vi "GDSLvClass_FlattenClass.vi"(0 "Class Refnum In":refnum<vi>, 3 "FlattenClass(T=>Flat,F=>Not Flat)":bool, 5 "error in (no error)":errorcluster) -> (14 "Class Refnum Out":refnum<vi>, 19 "error out":errorcluster)   [LabVIEW 2020]
panel:
  out "FoldersToActOn(Empty=>AllFolders) 2":string[](array[string])
  in  "FoldersToActOn(Empty=>AllFolders)":string[](array[string])
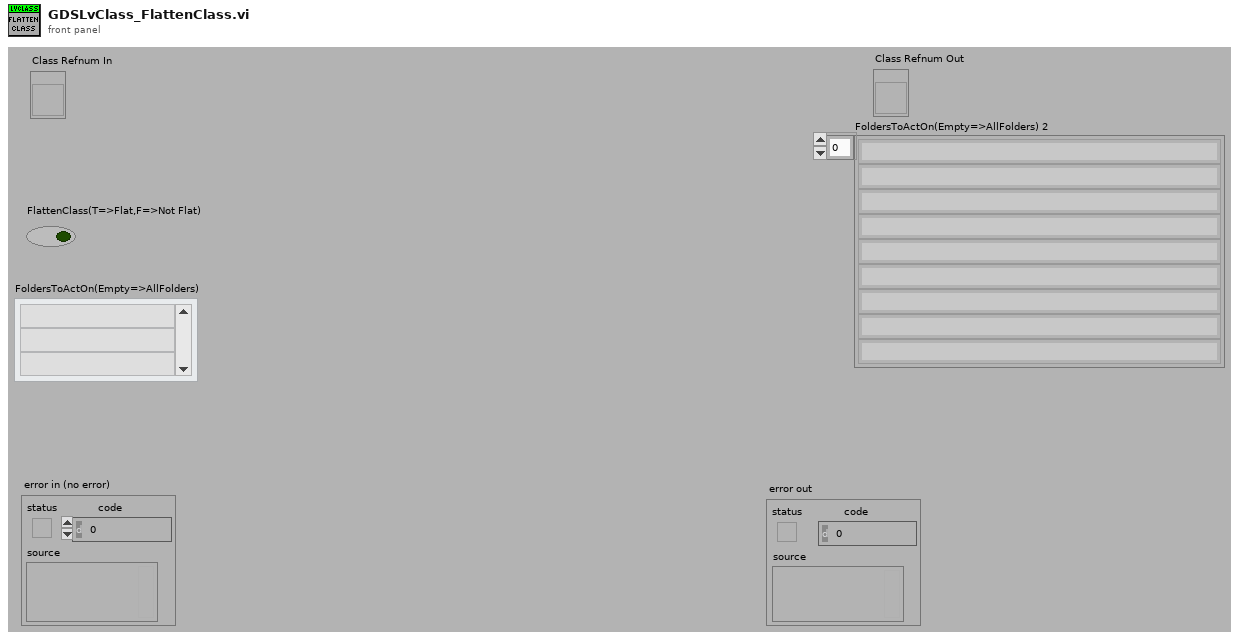
[diagram p1: front panel]
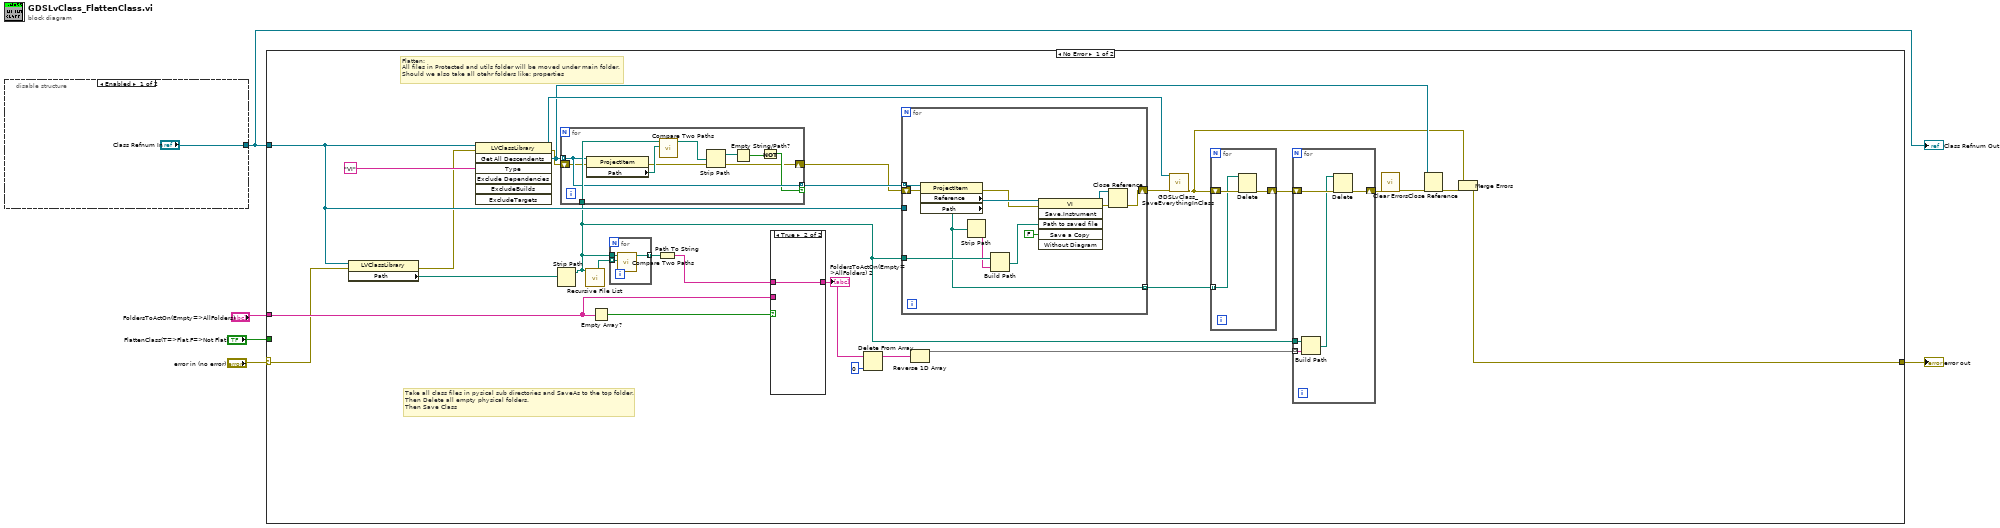
[diagram p0: block diagram]
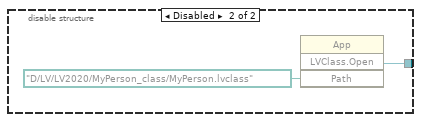
[diagram p2: hidden frame]
diagram:
  n1 = disable-structure shown="Enabled" {
    disable-tunnel: ["Class Refnum In" w8] -> w3
    frame Enabled {
    }
    frame Disabled {
      n2 = invoke class="App" method="LVClass.Open"("Path"=path "D:/LV/LV2020/MyPerson_class/MyPerson.lvclass") -> ("LVClass.Open"=w8:refnum<vi>)  [unwired: 3 in, 3 out]
    }
  }
  "Class Refnum Out" <- w3
  n3 = case shown="No Error" "error in (no error)" {
    selector: "error in (no error)" -> [w25 w71]
    tunnel: [w9 w71] -> w4
    tunnel: w3 -> [w28 _]
    tunnel: "FlattenClass(T=>Flat,F=>Not Flat)" -> [_ _]
    tunnel: "FoldersToActOn(Empty=>AllFolders)" -> [w33 _]
    frame No Error {
      # "Take all class files in pysical sub directories and SaveAs to the top folder.\nThen Delete all empty physical folders.\nThen Save Class"
      # "Flatten:\nAll files in Protected and utils folder will be moved under main folder.\nShould we also take all otehr folders like: properties"
      n4 = property class="LVClassLibrary"(reference=w28, error in=w25) -> (error out=w24:errorcluster, "Path"=w35:path)  [unwired: 1 out]
      n5 = invoke class="LVClassLibrary" method="Get All Descendents"(reference=w28, error in=w24, "Type"="VI") -> (reference out=w22:refnum<vi>, error out=w26:errorcluster, "All Descendents"=w12:refnum<vi>[])  [unwired: 4 in, 4 out]
      n6 = Strip Path(path=w35) -> (stripped path=w16:path)  [unwired: 1 out]
      n7 = for {
        tunnel: w12 -> [w60] mode=indexing
        tunnel: w16 -> [w65]
        tunnel: [w60] -> w29 mode=indexing if=w59
        shift-right: [w58] -> w27
        shift-left: w26 -> [w57]
        n8 = property class="ProjectItem"(reference=w60, error in=w57) -> (error out=w58:errorcluster, "Path"=w64:path)  [unwired: 1 out]
        n9 = call <vilib>:"Compare Two Paths.vi"("Path 2"=w64, "Path 1"=w65) -> ("Relative Path from 1 to 2"=w63:path)  [unwired: 6 in, 3 out]
        n10 = Strip Path(path=w63) -> (stripped path=w62:path)  [unwired: 1 out]
        n11 = Empty String/Path?(string/path=w62) -> (empty?=w61:bool)
        n12 = Not(x=w61) -> (.not. x?=w59:bool)
      }
      n13 = call <vilib>:"Recursive File List.vi"("Folder Path"=w16) -> ("All Folders"=w30:path[])  [unwired: 6 in, 4 out]
      n14 = Empty Array?(array=w33) -> (empty?=w34:bool)
      n15 = for {
        tunnel: w16 -> [w68]
        tunnel: w30 -> [w67] mode=indexing
        tunnel: [w66] -> w32 mode=indexing
        n16 = call <vilib>:"Compare Two Paths.vi"("Path 2"=w67, "Path 1"=w68) -> ("Relative Path from 1 to 2"=w66:path)  [unwired: 6 in, 3 out]
      }
      n17 = Path To String(path=w32) -> (string=w31:string[])
      n18 = case shown="True" w34 {
        tunnel: w31 -> [_ w70]
        tunnel: [w69 w70] -> w20
        tunnel: w33 -> [w69 _]
        frame False {
        }
        frame True {
        }
      }
      "FoldersToActOn(Empty=>AllFolders) 2" <- w20
      n19 = Delete From Array(array=w20, index=0) -> (array with subset deleted=w17:string[])  [unwired: 1 in, 1 out]
      n20 = for {
        tunnel: w29 -> [w56] mode=indexing
        tunnel: w28 -> [_]
        shift-right: [w46] -> w23
        shift-left: w27 -> [w55]
        tunnel: w16 -> [w52]
        tunnel: [w48] -> w21 mode=indexing
        n21 = property class="ProjectItem"(reference=w56, error in=w55) -> (error out=w53:errorcluster, "Reference"=w54:refnum<vi>, "Path"=w48:path)  [unwired: 1 out]
        n22 = Strip Path(path=w48) -> (name=w51:string)  [unwired: 1 out]
        n23 = Build Path(base path=w52, name or relative path=w51) -> (appended path=w50:path)
        n24 = invoke class="VI" method="Save.Instrument"(reference=w54, error in=w53, "Path to saved file"=w50, "Save a Copy"=FALSE) -> (reference out=w45:refnum<vi>, error out=w47:errorcluster)  [unwired: 2 in, 4 out]
        n25 = Close Reference(reference=w45, error in (no error)=w47) -> (error out=w46:errorcluster)
      }
      n26 = Reverse 1D Array(array=w17) -> (reversed array=w15:string[])
      n27 = call <resource>:"GDSLvClass_SaveEverythingInClass.vi"("ClassRefIn"=w22, "error in"=w23) -> ("error out"=w10:errorcluster)  [unwired: 16 in, 1 out]
      n28 = for {
        tunnel: w21 -> [w43] mode=indexing
        shift-right: [w42] -> w18
        shift-left: w10 -> [w44]
        n29 = Delete(path (use dialog)=w43, error in=w44) -> (error out=w42:errorcluster)  [unwired: 3 in, 2 out]
      }
      n30 = for {
        shift-right: [w40] -> w14
        shift-left: w18 -> [w41]
        tunnel: w16 -> [w39]
        tunnel: w15 -> [w38] mode=indexing
        n31 = Build Path(base path=w39, name or relative path=w38) -> (appended path=w37:path)
        n32 = Delete(path (use dialog)=w37, error in=w41) -> (error out=w40:errorcluster)  [unwired: 3 in, 2 out]
      }
      n33 = call <vilib>:"Clear Errors.vi"("error in (no error)"=w14) -> ("error out"=w13:errorcluster)  [unwired: 5 in, 1 out]
      n34 = Close Reference(reference=w12, error in (no error)=w13) -> (error out=w11:errorcluster)
      n35 = Merge Errors(w10, w11) -> (w9:errorcluster)
    }
    frame Error {
    }
  }
  "error out" <- w4
